vi "SC10_PIA_on_off_shutter_V2.vi"() -> ()   [LabVIEW 2010]
uses:
  <vilib>/DAQmx/read.llb/DAQmx Read (Analog 1D DBL 1Chan NSamp).vi
  <vilib>/DAQmx/create/channels.llb/DAQmx Create Channel (AI-Voltage-Basic).vi
  <vilib>/DAQmx/configure/timing.llb/DAQmx Timing (Sample Clock).vi
  <vilib>/daqmx/miscellaneous.llb/DAQmx Fill In Error Info.vi
panel:
  out "Iteration":i32
  out "iteration count":i32
  out "Average":dbl
  out "Model":string
  in  "Tab Control":enum32{"Setting", "Status", "Error Message"}(tab)
  in  "SC10 VISA":refnum<visa-resource-name>="COM3"
  in  "DAQ channels":tag="Dev1/ai4"
  in  "Data Bits":u16=8
  in  "Stop Bits":u16(ring)=10 items=["1.0"=10, "1.5"=15, "2.0"=20]
  in  "Flow Control":u16(ring) items=["None", "XON/XOFF", "RTS/CTS", "XON/XOFF & RTS/CTS", "DTR/DSR", "XON/XOFF & DTR/DSR"]
  in  "Baud Rate":u32=9600
  in  "Parity":u16(ring) items=["None", "Odd", "Even", "Mark", "Space"]
  in  "Mode":i32(ring)=1 items=["manual"=1, "auto"=2, "single"=3, "repeat"=4, "external gate"=5]
  in  "Trigger":i32(ring) items=["internal", "external"]
  out "Waveform Chart":dbl(graph)
  out "Trigger Status":bool
  out "Shutter Status":bool
  out "Counter":dbl
  out "Count":i32
  in  "Reset":bool
  in  "SC10 error in":errorcluster
  in  "DAQ error in":errorcluster
  out "DAQ error out":errorcluster
  out "SC10 VISA out":refnum<visa-resource-name>
  out "SC10 error out":errorcluster
  out "x/y":dbl
  in  "stop":bool
  # "Address Setting"
  # "SC10 Serial Setting"
  # "SC10 Setup Parameters\n\n- Baud Rate = 9600\n- Data Bits = 8\n- Parity = None\n- Stop Bits = 1\n- Flow Control = None"
  # "SC10 Setting"
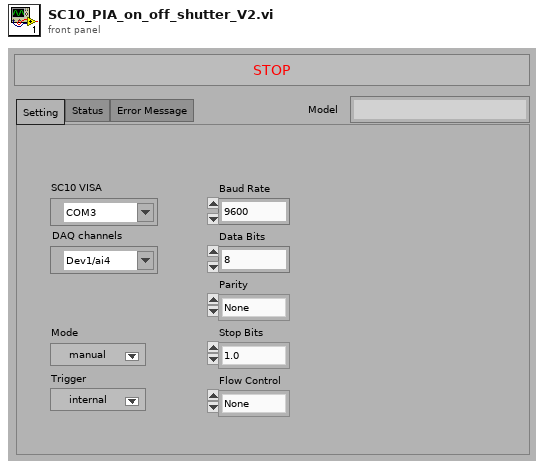
[diagram p1: front panel]
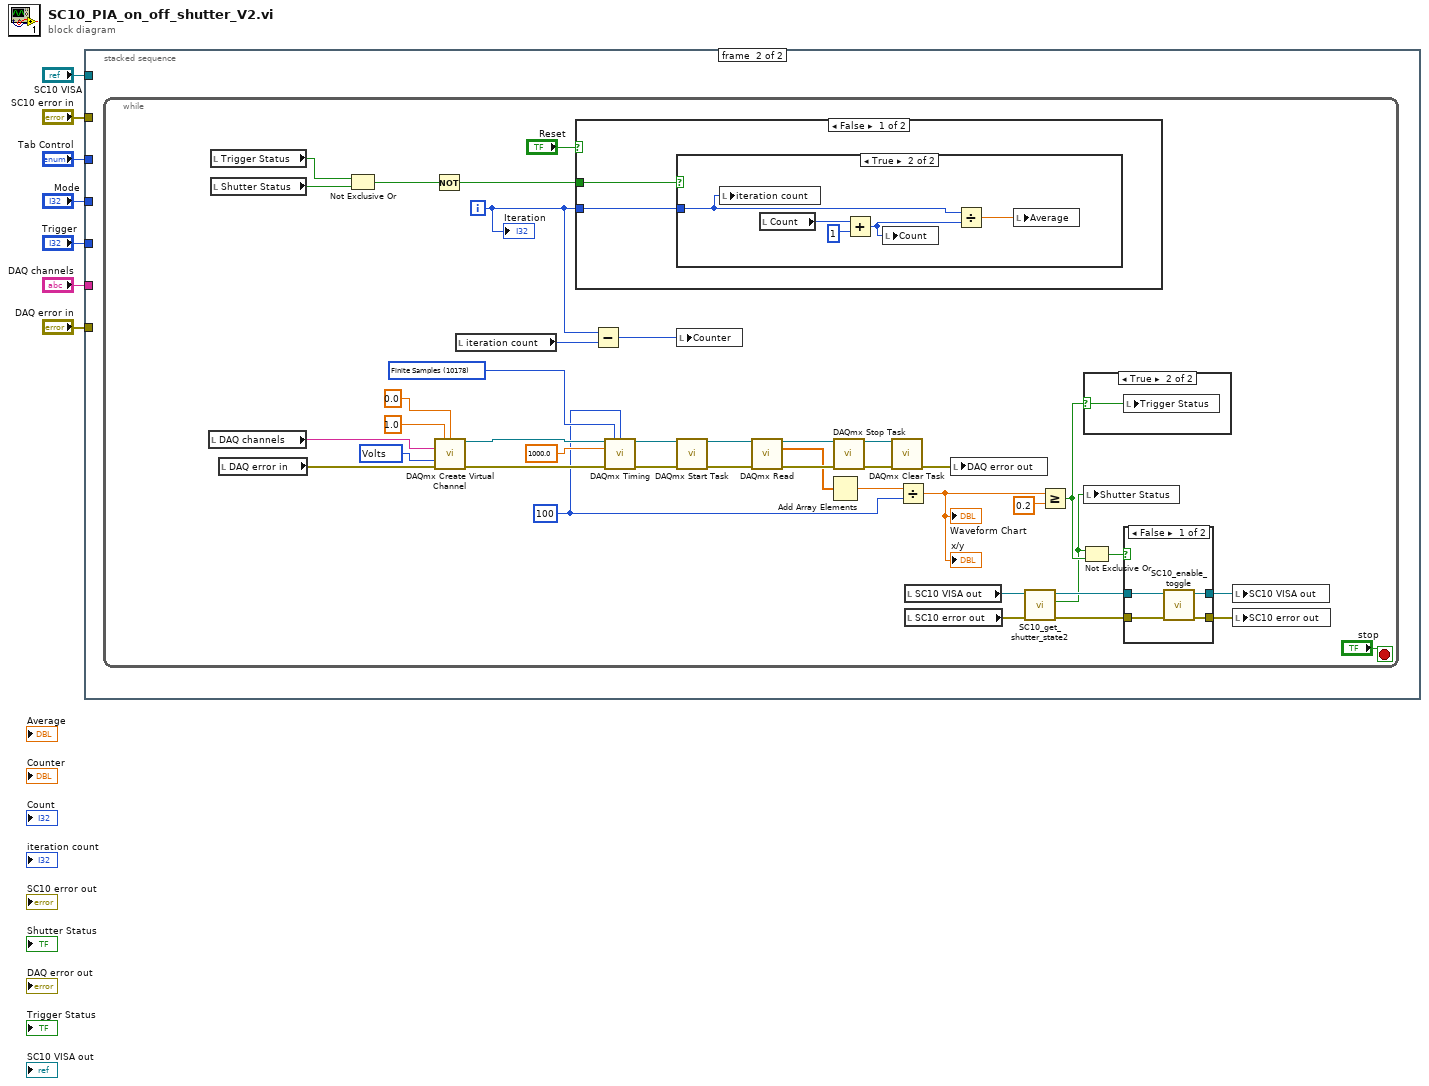
[diagram p0: block diagram]
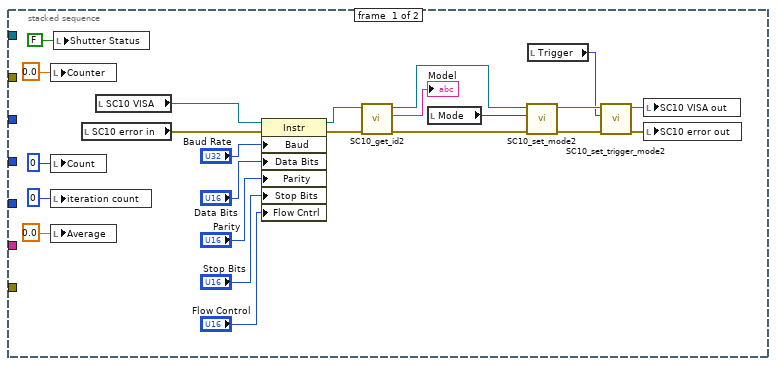
[diagram p2: hidden frame]
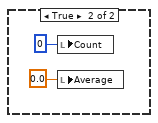
[diagram p4: hidden frame]
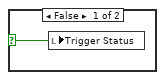
[diagram p5: hidden frame]
diagram:
  n1 = stacked-sequence {
    tunnel: "SC10 VISA" -> [_ _]
    tunnel: "SC10 error in" -> [_ _]
    tunnel: "Tab Control" -> [_ _]
    tunnel: "Mode" -> [_ _]
    tunnel: "Trigger" -> [_ _]
    tunnel: "DAQ channels" -> [_ _]
    tunnel: "DAQ error in" -> [_ _]
    frame #0 {
      n2 = local write "Counter"(0.0 ("Counter")) -> ()
      n3 = local write "Count"(0 ("Count")) -> ()
      n4 = local write "iteration count"(0 ("iteration count")) -> ()
      n5 = local write "Average"(0.0 ("Average")) -> ()
      n6 = local write "Shutter Status"(FALSE ("Shutter Status")) -> ()
      n7 = local read "SC10 error in"() -> (w19:errorcluster)
      n8 = local read "SC10 VISA"() -> (w21:refnum<visa-resource-name>)
      n9 = property class="Instr"(reference=w21, error in=w19, "Baud"="Baud Rate", "Data Bits"="Data Bits", "Parity"="Parity", "Stop Bits"="Stop Bits", "Flow Cntrl"="Flow Control") -> (reference out=w20:refnum<visa-resource-name>, error out=w18:errorcluster)
      n10 = call "SC10_get_id2.vi"("error in (no error)"=w18, "VISA resource name"=w20) -> ("error out"=w28:errorcluster, "Model"=→"Model":string, "VISA resource name out"=w27:refnum<visa-resource-name>)  [unwired: 7 in]
      n11 = local read "Mode"() -> (w23:i32)
      n12 = call "SC10_set_mode2.vi"("error in (no error)"=w28, "mode"=w23, "VISA resource name"=w27) -> ("error out"=w29:errorcluster, "VISA resource name out"=w30:refnum<visa-resource-name>)  [unwired: 5 in]
      n13 = local read "Trigger"() -> (w22:i32)
      n14 = call "SC10_set_trigger_mode2.vi"("error in (no error)"=w29, "trigger mode"=w22, "VISA resource name"=w30) -> ("error out"=w25:errorcluster, "VISA resource name out"=w24:refnum<visa-resource-name>)  [unwired: 7 in]
      n15 = local write "SC10 VISA out"(w24) -> ()
      n16 = local write "SC10 error out"(w25) -> ()
    }
    frame #1 {
      n17 = while {
        i -> [w33]
        stop <- "stop" stop-if-true
        w50 = 100 ("samples per channel")
        w62 = 10178 items=["Finite Samples"=10178, "Continuous Samples"=10123, "Hardware Timed Single Point"=12522] ("sample mode")
        w68 = 10348 items=["Volts"=10348, "From Custom Scale"=10065] ("units")
        n18 = local read "DAQ channels"() -> (w46:tag)
        n19 = local read "Trigger Status"() -> (w34:bool)
        n20 = local read "Shutter Status"() -> (w37:bool)
        n21 = local read "DAQ error in"() -> (w47:errorcluster)
        n22 = Not Exclusive Or(1:w37, 2:w34) -> (0:w36:bool)
        n23 = Not(x=w36) -> (.not. x?=w35:bool)
        n24 = call-poly <vilib>:"DAQmx Create Virtual Channel.vi"("maximum value"=1.0, "minimum value"=0.0, "physical channels"=w46, "units"=w68, "error in"=w47) -> ("task out"=w65:refnum<k21>, "error out"=w64:errorcluster)  [unwired: 4 in, 5 out]
        n25 = local read "iteration count"() -> (w39:i32)
        n26 = case shown="False" "Reset" {
          tunnel: w35 -> [w72 _]
          tunnel: w33 -> [w73 _]
          frame False {
            n27 = case shown="True" w72 {
              tunnel: w73 -> [_ w78]
              frame False {
              }
              frame True {
                n28 = local write "iteration count"(w78) -> ()
                n29 = local read "Count"() -> (w77:i32)
                n30 = Add(x=w77, y=1) -> (x+y=w75:i32)
                n31 = local write "Count"(w75) -> ()
                n32 = Divide(x=w78, y=w75) -> (x/y=w74:dbl)
                n33 = local write "Average"(w74) -> ()
              }
            }
          }
          frame True {
            n34 = local write "Count"(0 ("Count")) -> ()
            n35 = local write "Average"(0.0 ("Average")) -> ()
          }
        }
        n36 = Subtract(x=w33, y=w39) -> (x-y=w38:i32)
        n37 = call-poly <vilib>:"DAQmx Timing.vi"("task/channels in"=w65, "sample mode"=w62, "samples per channel"=w50, "rate"=1000.0, "error in"=w64) -> ("task out"=w61:refnum<k21>, "error out"=w60:errorcluster)  [unwired: 2 in, 7 out]
        n38 = local write "Counter"(w38) -> ()
        n39 = call <vilib>:"DAQmx Start Task.vi"("task/channels in"=w61, "error in"=w60) -> ("task out"=w59:refnum<k21>, "error out"=w58:errorcluster)  [unwired: 12 out]
        n40 = call-poly <vilib>:"DAQmx Read.vi"("task/channels in"=w59, "error in"=w58) -> ("task out"=w56:refnum<k21>, "data"=w52:dbl[], "error out"=w55:errorcluster)  [unwired: 1 in, 10 out]
        n41 = Add Array Elements(numeric array=w52) -> (sum=w51:dbl)
        n42 = call <vilib>:"DAQmx Stop Task.vi"("task/channels in"=w56, "error in"=w55) -> ("task out"=w54:refnum<k21>, "error out"=w53:errorcluster)  [unwired: 12 out]
        n43 = call <vilib>:"DAQmx Clear Task.vi"("task in"=w54, "error in"=w53) -> ("error out"=w40:errorcluster)  [unwired: 13 out]
        n44 = Divide(x=w51, y=w50) -> (x/y=w48:dbl)
        "x/y" <- w48
        "Waveform Chart" <- w48
        n45 = local read "SC10 VISA out"() -> (w43:refnum<visa-resource-name>)
        n46 = local read "SC10 error out"() -> (w44:errorcluster)
        n47 = local write "DAQ error out"(w40) -> ()
        n48 = call "SC10_get_shutter_state2.vi"("error in (no error)"=w44, "VISA resource name"=w43) -> ("error out"=w71:errorcluster, "open(true)"=w41:bool, "VISA resource name out"=w70:refnum<visa-resource-name>)  [unwired: 6 in, 1 out]
        n49 = Greater Or Equal?(x=w48, y=0.2) -> (x >= y?=w49:bool)
        n50 = Not Exclusive Or(1:w49, 2:w41) -> (0:w69:bool)
        n51 = case shown="True" w49 {
          selector: w49 -> [w81 w82]
          frame False {
            n52 = local write "Trigger Status"(w81) -> ()
          }
          frame True {
            n53 = local write "Trigger Status"(w82) -> ()
          }
        }
        n54 = local write "Shutter Status"(w41) -> ()
        n55 = case shown="False" w69 {
          tunnel: w71 -> [w86 w87]
          tunnel: w70 -> [w85 w88]
          tunnel: [w84 w88] -> w42
          tunnel: [w83 w87] -> w45
          frame False {
            n56 = call "SC10_enable_toggle.vi"("error in (no error)"=w86, "VISA resource name"=w85) -> ("error out"=w83:errorcluster, "VISA resource name out"=w84:refnum<visa-resource-name>)  [unwired: 8 in]
          }
          frame True {
          }
        }
        n57 = local write "SC10 VISA out"(w42) -> ()
        n58 = local write "SC10 error out"(w45) -> ()
        "Iteration" <- w33
      }
    }
  }
